vi "GFITS_GetImageParams.vi"(9 "defexts":bool=TRUE, 11 "Database RefNum":T1) -> (2 "imageStruct":T2={"name"="/home/bonati/images/mono022", "Path"=path "", "bitpix"=16, "naxis"=2, "naxes"=[2224, 2048], "datatype"=0, "multiple extensions"=FALSE, "hdutype"=0, "writeToDisk"=TRUE, "num_of_ext"=0, "file ref"=0, "createnewimage"=TRUE}, 4 "CurrentReadMode":string, 5 "header template":path=path "/home/ArcVIEW/ConfigFile/hdr.ir", 6 "totele":u32)   [LabVIEW 2016]
uses:
  DBSHAND/private/vis/DatabaseHand_RefNum.ctl
  DBSHAND/private/vis/DatabaseHand_Element_Get(bool).vi
  DBSHAND/private/vis/DatabaseHand_Element_Get(I32).vi
  DBSHAND/private/vis/DatabaseHand_Element_Get(string).vi
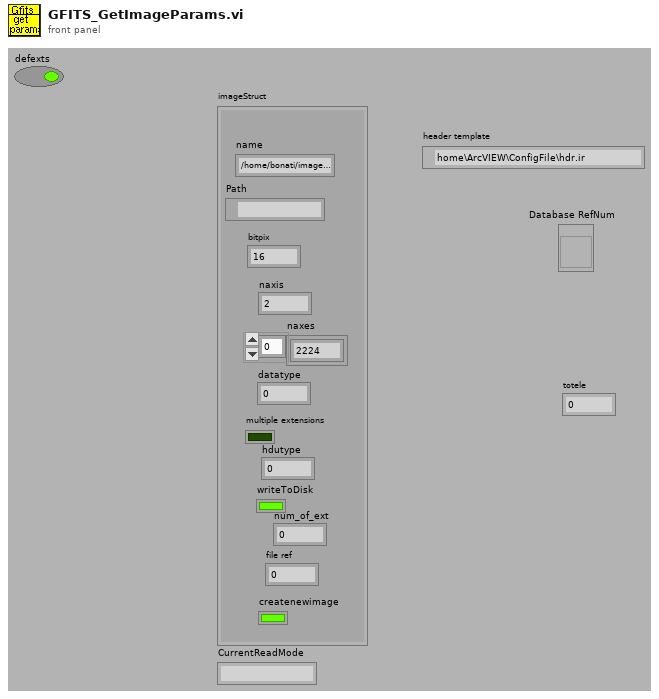
[diagram p1: front panel]
types:
  T1 = typedef "DatabaseHand_RefNum.ctl" = refnum<vi>
  T2 = cluster{"name":string, "Path":path, "bitpix":i8, "naxis":u8, "naxes":u32[], "datatype":u16, "multiple extensions":bool, "hdutype":u16, "writeToDisk":bool, "num_of_ext":u8, "file ref":i32, "createnewimage":bool}
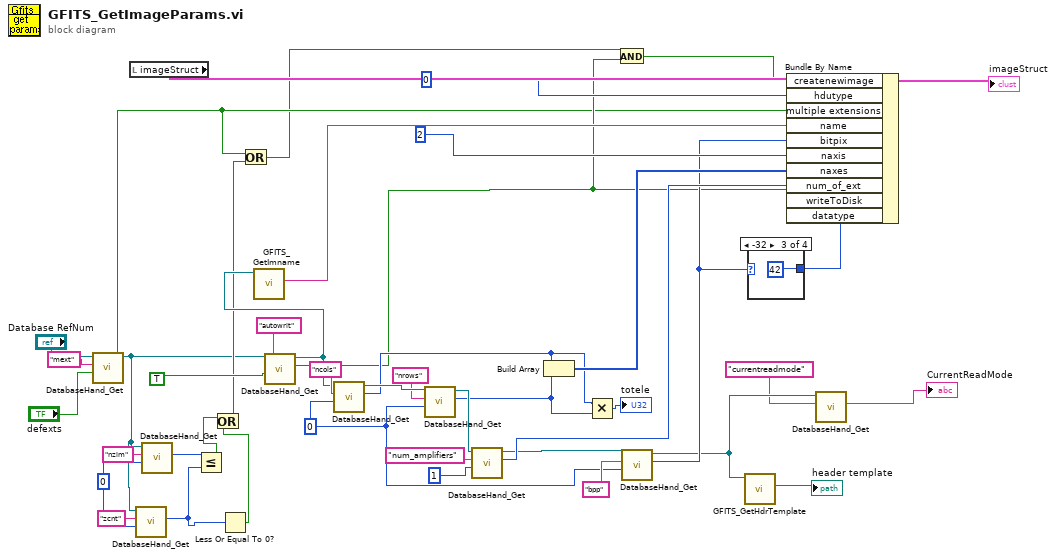
[diagram p0: block diagram]
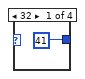
[diagram p2: hidden frame]
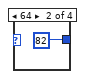
[diagram p3: hidden frame]
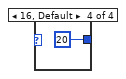
[diagram p4: hidden frame]
diagram:
  w4 = 0
  w23 = 0
  n1 = call-poly "DatabaseHand_Get.vi"("default value"="defexts", "name"="mext", "Database RefNum in"="Database RefNum") -> ("value"=w11:bool, "Database RefNum out"=w6:T1)  [unwired: 2 in, 5 out]
  n2 = local read "imageStruct"() -> (w44:T2)
  n3 = call-poly "DatabaseHand_Get.vi"("default value"=w4, "name"="zcnt", "Database RefNum in"=w6) -> ("value"=w3:i32)  [unwired: 2 in, 6 out]
  n4 = call-poly "DatabaseHand_Get.vi"("default value"=w4, "name"="nzim", "Database RefNum in"=w6) -> ("value"=w14:i32)  [unwired: 2 in, 6 out]
  n5 = Less Or Equal?(x=w14, y=w3) -> (x <= y?=w8:bool)
  n6 = Less Or Equal To 0?(x=w3) -> (x <= 0?=w7:bool)
  n7 = Or(x=w8, y=w7) -> (x .or. y?=w9:bool)
  n8 = Or(x=w11, y=w9) -> (x .or. y?=w10:bool)
  n9 = call-poly "DatabaseHand_Get.vi"("default value"=TRUE, "name"="autowrit", "Database RefNum in"=w6) -> ("value"=w12:bool, "Database RefNum out"=w30:T1)  [unwired: 2 in, 5 out]
  n10 = call "GFITS_GetImname.vi"("Database RefNum"=w30) -> ("name"=w34:string)  [unwired: 10 out]
  n11 = call-poly "DatabaseHand_Get.vi"("default value"=w23, "name"="ncols", "Database RefNum in"=w30) -> ("value"=w21:i32, "Database RefNum out"=w33:T1)  [unwired: 2 in, 5 out]
  n12 = call-poly "DatabaseHand_Get.vi"("default value"=w23, "name"="nrows", "Database RefNum in"=w33) -> ("value"=w20:i32, "Database RefNum out"=w29:T1)  [unwired: 2 in, 5 out]
  n13 = call-poly "DatabaseHand_Get.vi"("default value"=1, "name"="num_amplifiers", "Database RefNum in"=w29) -> ("value"=w27:i32, "Database RefNum out"=w26:T1)  [unwired: 2 in, 5 out]
  n14 = Build Array(w21, w20) -> (w39:i32[])
  n15 = Multiply(x=w21, y=w20) -> (x*y=→"totele":i32)
  n16 = And(x=w10, y=w12) -> (x .and. y?=w13:bool)
  n17 = call-poly "DatabaseHand_Get.vi"("default value"=w23, "name"="bpp", "Database RefNum in"=w26) -> ("value"=w24:i32, "Database RefNum out"=w18:T1)  [unwired: 2 in, 5 out]
  n18 = call "GFITS_GetHdrTemplate.vi"("Database RefNum"=w18) -> ("path"=→"header template":path)  [unwired: 10 out]
  n19 = case shown="-32" w24 {
    tunnel: [41 82 42 20] -> w40
    frame 32 {
    }
    frame 64 {
    }
    frame -32 {
    }
    frame 16, Default {
    }
  }
  n20 = Bundle By Name(cluster=w44, "createnewimage"=w13, "hdutype"=u16 0, "multiple extensions"=w11, "name"=w34, "bitpix"=w24, "naxis"=u8 2, "naxes"=w39, "num_of_ext"=w27, "writeToDisk"=w12, "datatype"=w40) -> (→"imageStruct":T2)
  n21 = call-poly "DatabaseHand_Get.vi"("name"="currentreadmode", "Database RefNum in"=w18) -> ("value"=→"CurrentReadMode":string)  [unwired: 3 in, 6 out]
